vi "Set Command Handling.vi"(8 "error in (no error)":errorcluster, 11 "Disable Command Handling":bool) -> (0 "error out":errorcluster)   [LabVIEW 2017, in "Command Handler.lvlib"]
uses:
  Command Handler.lvlib
  Command Handler Global.vi
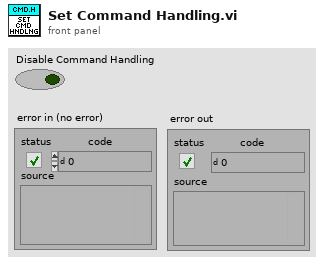
[diagram p1: front panel]
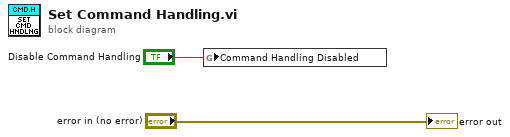
[diagram p0: block diagram]
diagram:
  n1 = global write "Command Handler Global.vi" "Command Handling Disabled"("Disable Command Handling") -> ()
  "error out" <- "error in (no error)"
